vi "CBL Close Device.vi"(11 "DevIndex":i32) -> (3 "function return":i32)   [LabVIEW 2010, in "CANBootloader.lvlib"]
doc: "int WINAPI CBL_CloseDevice(int DevIndex);"
uses:
  CANBootloader.lvlib
  CANBootloader/Ginkgo_Driver.dll
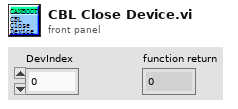
[diagram p1: front panel]
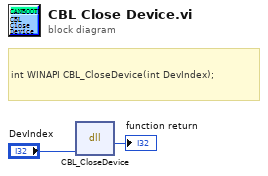
[diagram p0: block diagram]
diagram:
  # "int WINAPI CBL_CloseDevice(int DevIndex);"
  n1 = dll-call lib="E:/Project/vt_ginkgo/truck/Ginkgo Driver/vs2010/Ginkgo_USB-I2C&SPI&CAN_API_v2.0.3.3/lib/labview_32bit/CANBootloader/Ginkgo_Driver.*" fn="CBL_CloseDevice"("DevIndex"="DevIndex") -> (→"function return":i32)  [unwired: 4 in, 2 out]
